vi "readFromXML.vi"(8 "error in (no error)":errorcluster, 10 "XML in":string="  <AOSPointingOffset>\n\t\t<xCorrection_arcsec>66</xCorrection_arcsec>\n\t\t<yCorrection_arcsec>55</yCorrection_arcsec>\n  </AOSPointingOffset>", 11 "AOSPointingOffset.lvclass":refnum<class "AOSPointingOffset.lvclass">) -> (0 "error out":errorcluster, 3 "AOSPointingOffset.lvclass 2":refnum<class "AOSPointingOffset.lvclass">)   [LabVIEW 2022 SP3, in "TCSDataDefinitions.lvlib" / "TCSActiveOpticsCommand.lvlib" / "AOSPointingOffset.lvclass"]
uses:
  AOSPointingOffset.lvclass
  <userlib>/Common/UnitsAndXML/FlattenItemWithUnitToXML/FlattenPlaneAngleToXML/PlaneAngleUnit.ctl
  AOSPointingOffset.lvclass/AOSPointingOffset.ctl
  TCSActiveOpticsCommand/TCSActiveOpticsCommand.lvclass
  <userlib>/Common/UnitsAndXML/UnitsAndXML.lvlib
  <userlib>/Common/XML/XMLParser/XMLParser.lvclass
panel:
  out "xCorrection_arcsec":dbl[unit]=0.00031997702953229375
  out "yCorrrection_arcsec":dbl[unit]=0.0002666475246102448
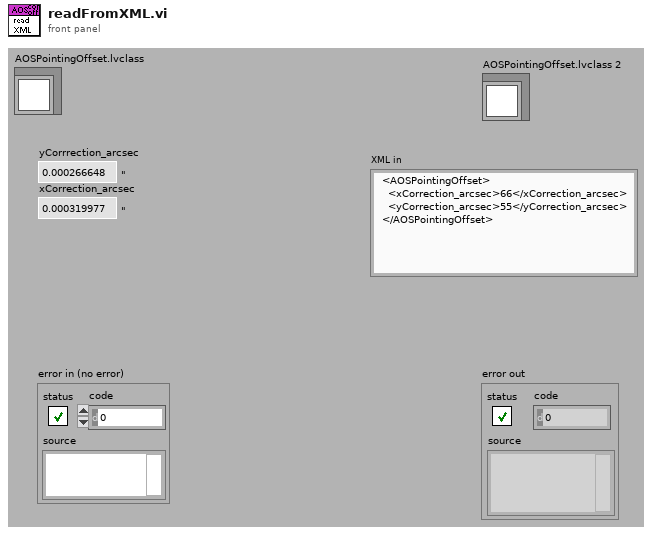
[diagram p1: front panel]
types:
  T1 = typedef "UnitsAndXML.lvlib/PlaneAngleUnit.ctl" = enum16{"rad", "deg", "'", "\""}
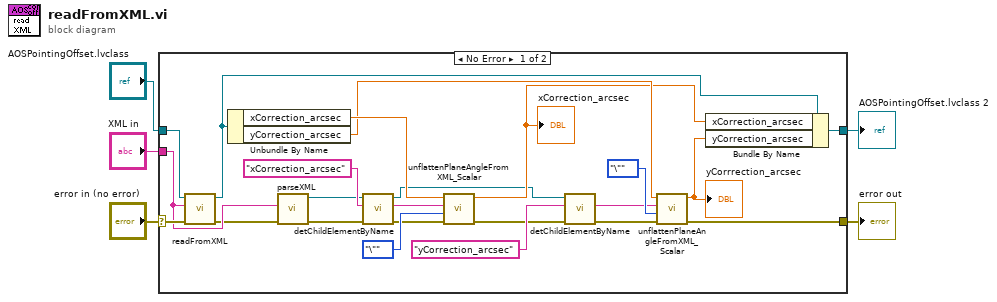
[diagram p0: block diagram]
diagram:
  n1 = case shown="No Error" "error in (no error)" {
    selector: "error in (no error)" -> [w26 w30]
    tunnel: [w19 w30] -> w4
    tunnel: [w28 w29] -> w3
    tunnel: "AOSPointingOffset.lvclass" -> [w27 w29]
    tunnel: "XML in" -> [w17 _]
    frame No Error {
      n2 = call-parent "readFromXML.vi"("error in (no error)"=w26, "XML in"=w17, "TCSActiveOpticsCommand in"=w27) -> ("error out"=w15:errorcluster, "TCSActiveOpticsCommand out"=w25:refnum<class "AOSPointingOffset.lvclass">)  [unwired: 7 out]
      n3 = Unbundle By Name(w25) -> ("xCorrection_arcsec"=w24:dbl[unit], "yCorrection_arcsec"=w22:dbl[unit])
      n4 = call <userlib>:"parseXML.vi"("error in (no error)"=w15, "XMLString in"=w17) -> ("error out"=w16:errorcluster, "Element out"=w10:refnum<class "XMLParser.lvclass">)  [unwired: 8 in]
      n5 = call <userlib>:"detChildElementByName.vi"("error in (no error)"=w16, "childName"="xCorrection_arcsec" ("ChildName"), "Element in"=w10) -> ("error out"=w8:errorcluster, "childXML"=w14:string, "Element out"=w6:refnum<class "XMLParser.lvclass">)  [unwired: 5 in, 1 out]
      n6 = call <userlib>:"unflattenPlaneAngleFromXML_Scalar.vi"("error in (no error)"=w8, "planeAngleUnitInXML"=PlaneAngleUnit."\"", "xmlString"=w14, "planeAngleForType"=w24) -> ("error out"=w7:errorcluster, "planeAngle"=w20:dbl[unit])  [unwired: 6 in]
      "xCorrection_arcsec" <- w20
      n7 = call <userlib>:"detChildElementByName.vi"("error in (no error)"=w7, "childName"="yCorrection_arcsec" ("ChildName"), "Element in"=w6) -> ("error out"=w9:errorcluster, "childXML"=w12:string)  [unwired: 5 in, 2 out]
      n8 = call <userlib>:"unflattenPlaneAngleFromXML_Scalar.vi"("error in (no error)"=w9, "planeAngleUnitInXML"=PlaneAngleUnit."\"", "xmlString"=w12, "planeAngleForType"=w22) -> ("error out"=w19:errorcluster, "planeAngle"=w11:dbl[unit])  [unwired: 6 in]
      "yCorrrection_arcsec" <- w11
      n9 = Bundle By Name(cluster=w25, "xCorrection_arcsec"=w20, "yCorrection_arcsec"=w11) -> (w28:refnum<class "AOSPointingOffset.lvclass">)
    }
    frame Error {
    }
  }
  "error out" <- w4
  "AOSPointingOffset.lvclass 2" <- w3
